vi "LightIndicators (SubVI).vi"(9 "State [GYBWR]":bool[](array[boolean]), 10 "Indicators [GYBWR]":refnum<vi>) -> ()   [LabVIEW 2014]
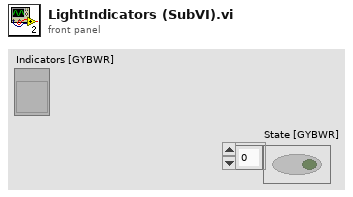
[diagram p1: front panel]
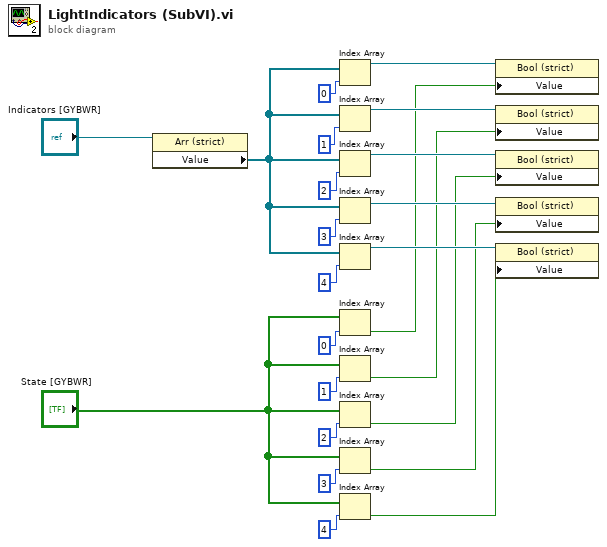
[diagram p0: block diagram]
diagram:
  n1 = property class="Arr (strict)"(reference="Indicators [GYBWR]") -> ("Value"=w2:refnum<vi>[])  [unwired: 1 in, 2 out]
  n2 = Index Array(array=w2, index=0) -> (element=w16:refnum<vi>)
  n3 = Index Array(array=w2, index=1) -> (element=w15:refnum<vi>)
  n4 = Index Array(array=w2, index=2) -> (element=w14:refnum<vi>)
  n5 = Index Array(array=w2, index=3) -> (element=w13:refnum<vi>)
  n6 = Index Array(array=w2, index=4) -> (element=w12:refnum<vi>)
  n7 = Index Array(array="State [GYBWR]", index=0) -> (element=w6:bool)
  n8 = Index Array(array="State [GYBWR]", index=1) -> (element=w1:bool)
  n9 = Index Array(array="State [GYBWR]", index=2) -> (element=w5:bool)
  n10 = Index Array(array="State [GYBWR]", index=3) -> (element=w4:bool)
  n11 = Index Array(array="State [GYBWR]", index=4) -> (element=w3:bool)
  n12 = property class="Bool (strict)"(reference=w16, "Value"=w6) -> ()  [unwired: 1 in, 2 out]
  n13 = property class="Bool (strict)"(reference=w15, "Value"=w1) -> ()  [unwired: 1 in, 2 out]
  n14 = property class="Bool (strict)"(reference=w14, "Value"=w5) -> ()  [unwired: 1 in, 2 out]
  n15 = property class="Bool (strict)"(reference=w13, "Value"=w4) -> ()  [unwired: 1 in, 2 out]
  n16 = property class="Bool (strict)"(reference=w12, "Value"=w3) -> ()  [unwired: 1 in, 2 out]
